vi "GetParameterInfo.vi"(7 "Camera Parameter":T2, 8 "error in (no error)":errorcluster, 11 "Stream":refnum<data-value>) -> (0 "error out":errorcluster, 2 "Info":T1, 3 "Stream (duplicate)":refnum<data-value>)   [LabVIEW 2020, in "g_ar_toolkit.capture.lvlib" / "CameraStream.lvclass"]
uses:
  CameraStream.lvclass
  Camera Parameters.ctl
  Camera Parameter Information.ctl
  CameraStream.lvclass/CameraStream.ctl
  bin/g_ar_toolkit.1.32.dll
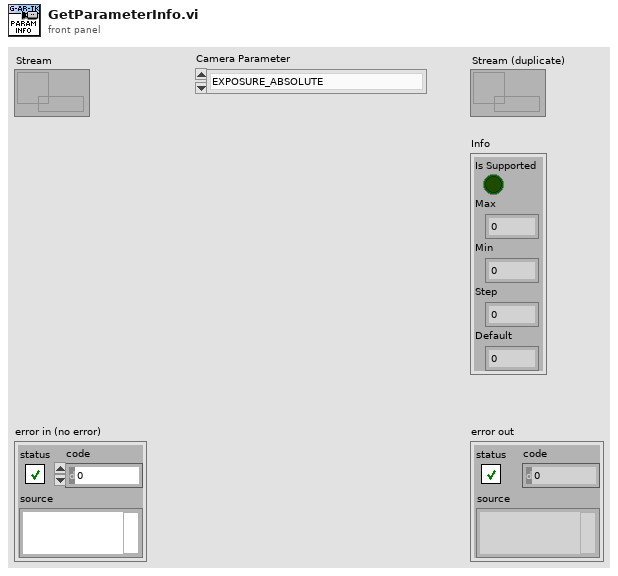
[diagram p1: front panel]
types:
  T1 = typedef "g_ar_toolkit.capture.lvlib/CameraStream.lvclass/Camera Parameter Information.ctl" = cluster{"Is Supported":bool, "Max":i32, "Min":i32, "Step":i32, "Default":i32}
  T2 = typedef "g_ar_toolkit.capture.lvlib/CameraStream.lvclass/Camera Parameters.ctl" = enum8{"EXPOSURE_ABSOLUTE", "FOCUS_ABSOLUTE", "ZOOM_ABSOLUTE", "WHITE_BALANCE_TEMPERATURE", "BRIGHTNESS", "CONTRAST", "SATURATION", "GAMMA", "HUE", "SHARPNESS", "BACKLIGHT_COMPENSATION", "POWER_LINE_FREQUENCY"}
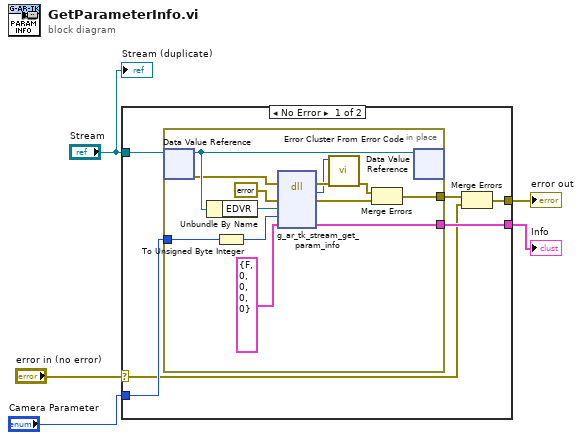
[diagram p0: block diagram]
diagram:
  n1 = case shown="No Error" "error in (no error)" {
    selector: "error in (no error)" -> [w6 w25]
    tunnel: [w9 w25] -> w4
    tunnel: "Stream" -> [w10 _]
    tunnel: "Camera Parameter" -> [w8 _]
    tunnel: [w7 _] -> w1
    frame No Error {
      n2 = in-place {
        in-place-border: [w24] -> w11
        in-place-border: w8 -> [w15]
        in-place-border: [w13] -> w7
        n3 = in-place-dvr #1(w10) -> (w22:refnum<class "CameraStream.lvclass">, w21:errorcluster)
        n4 = Unbundle By Name(w22) -> ("EDVR"=w23:refnum<data-value>)
        n5 = To Unsigned Byte Integer(number=w15) -> (unsigned 8bit integer=w12:u8)
        n6 = dll-call lib="C:/serenial/libraries/g-augmented-reality-toolkit/LabVIEW/bin/g_ar_toolkit.1.*.*" fn="g_ar_tk_stream_get_param_info" ("g_ar_toolkit.*.*:g_ar_tk_stream_capture_next")(error in=w21, "error_cluster"=errorcluster {"status"=FALSE, "code"=0, "source"=""} ("error constant"), "EDVR_strm"=w23, "parameter"=w12, "info"=T1 {"Is Supported"=FALSE, "Max"=0, "Min"=0, "Step"=0, "Default"=0} ("Camera Parameter Information")) -> (error out=w20:errorcluster, "MgErr"=w19:i32, "error_cluster"=w17:errorcluster, "info"=w13:T1)  [unwired: 4 in, 1 out]
        n7 = call <vilib>:"Error Cluster From Error Code.vi"("error in (no error)"=w20, "error code (0)"=w19) -> ("error out"=w18:errorcluster)  [unwired: 7 in]
        n8 = Merge Errors(w18, w17) -> (w24:errorcluster)
        n9 = in-place-dvr #1(w22) -> ()  [unwired: 2 out]
      }
      n10 = Merge Errors(w11, w6) -> (w9:errorcluster)
    }
    frame Error {
    }
  }
  "error out" <- w4
  "Info" <- w1
  "Stream (duplicate)" <- "Stream"
